vi "VCI_BOARD_INFO_1_CONVERT.vi"(1 "VCI_BOARD_INFO_1":T2) -> (0 "VCI_BOARD_INFO":T1)   [LabVIEW 2018, in "ControlCan.lvlib"]
uses:
  ControlCan.lvlib
  VCI_BOARD_INFO_1.ctl
  VCI_BOARD_INFO.ctl
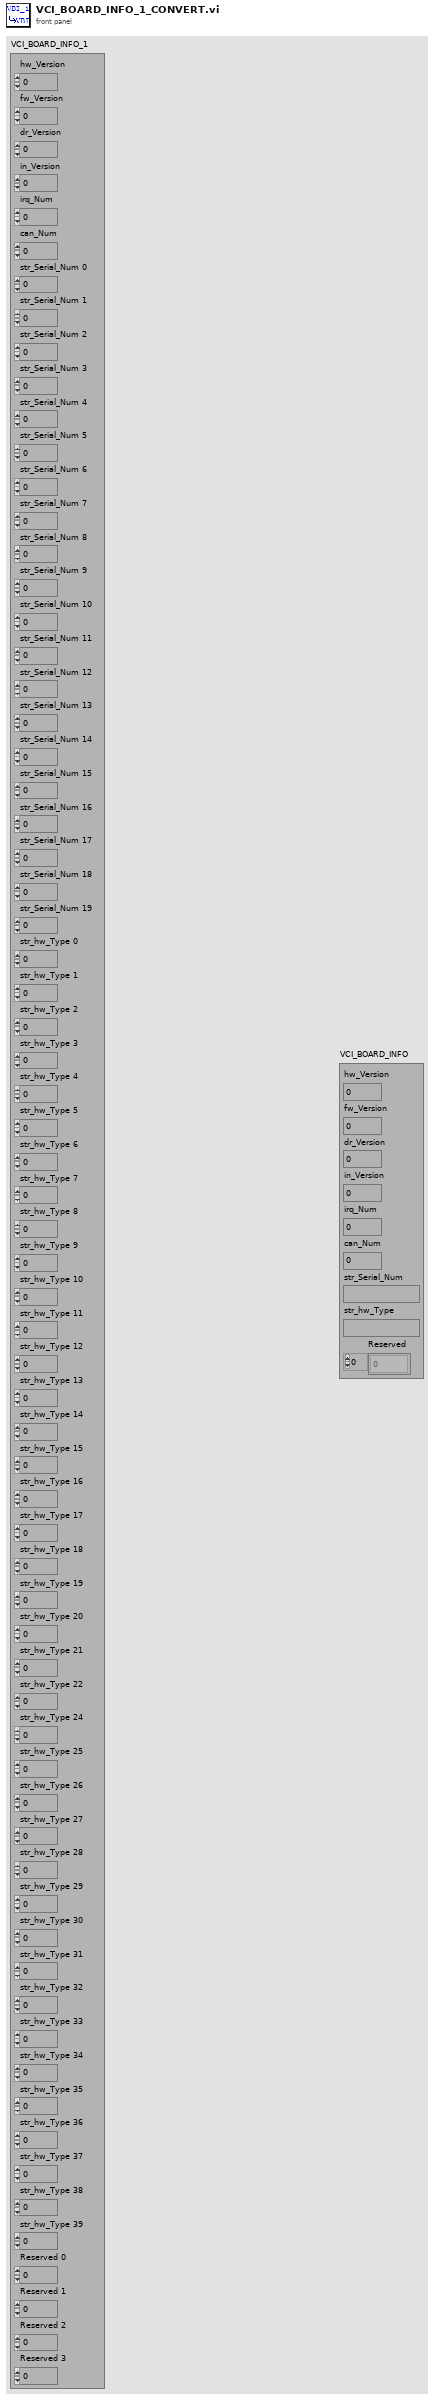
[diagram p1: front panel]
types:
  T1 = typedef "ControlCAN.lvlib/VCI_BOARD_INFO.ctl" = cluster{"hw_Version":u16, "fw_Version":u16, "dr_Version":u16, "in_Version":u16, "irq_Num":u16, "can_Num":u8, "str_Serial_Num":string, "str_hw_Type":string, "Reserved":u8[]}
  T2 = typedef "ControlCAN.lvlib/VCI_BOARD_INFO_1.ctl" = cluster{"hw_Version":u16, "fw_Version":u16, "dr_Version":u16, "in_Version":u16, "irq_Num":u16, "can_Num":u8, "str_Serial_Num 0":u8, "str_Serial_Num 1":u8, "str_Serial_Num 2":u8, "str_Serial_Num 3":u8, "str_Serial_Num 4":u8, "str_Serial_Num 5":u8, "str_Serial_Num 6":u8, "str_Serial_Num 7":u8, "str_Serial_Num 8":u8, "str_Serial_Num 9":u8, "str_Serial_Num 10":u8, "str_Serial_Num 11":u8, "str_Serial_Num 12":u8, "str_Serial_Num 13":u8, "str_Serial_Num 14":u8, "str_Serial_Num 15":u8, "str_Serial_Num 16":u8, "str_Serial_Num 17":u8, "str_Serial_Num 18":u8, "str_Serial_Num 19":u8, "str_hw_Type 0":u8, "str_hw_Type 1":u8, "str_hw_Type 2":u8, "str_hw_Type 3":u8, "str_hw_Type 4":u8, "str_hw_Type 5":u8, "str_hw_Type 6":u8, "str_hw_Type 7":u8, "str_hw_Type 8":u8, "str_hw_Type 9":u8, "str_hw_Type 10":u8, "str_hw_Type 11":u8, "str_hw_Type 12":u8, "str_hw_Type 13":u8, "str_hw_Type 14":u8, "str_hw_Type 15":u8, "str_hw_Type 16":u8, "str_hw_Type 17":u8, "str_hw_Type 18":u8, "str_hw_Type 19":u8, "str_hw_Type 20":u8, "str_hw_Type 21":u8, "str_hw_Type 22":u8, "str_hw_Type 24":u8, "str_hw_Type 25":u8, "str_hw_Type 26":u8, "str_hw_Type 27":u8, "str_hw_Type 28":u8, "str_hw_Type 29":u8, "str_hw_Type 30":u8, "str_hw_Type 31":u8, "str_hw_Type 32":u8, "str_hw_Type 33":u8, "str_hw_Type 34":u8, "str_hw_Type 35":u8, "str_hw_Type 36":u8, "str_hw_Type 37":u8, "str_hw_Type 38":u8, "str_hw_Type 39":u8, "Reserved 0":u8, "Reserved 1":u8, "Reserved 2":u8, "Reserved 3":u8}
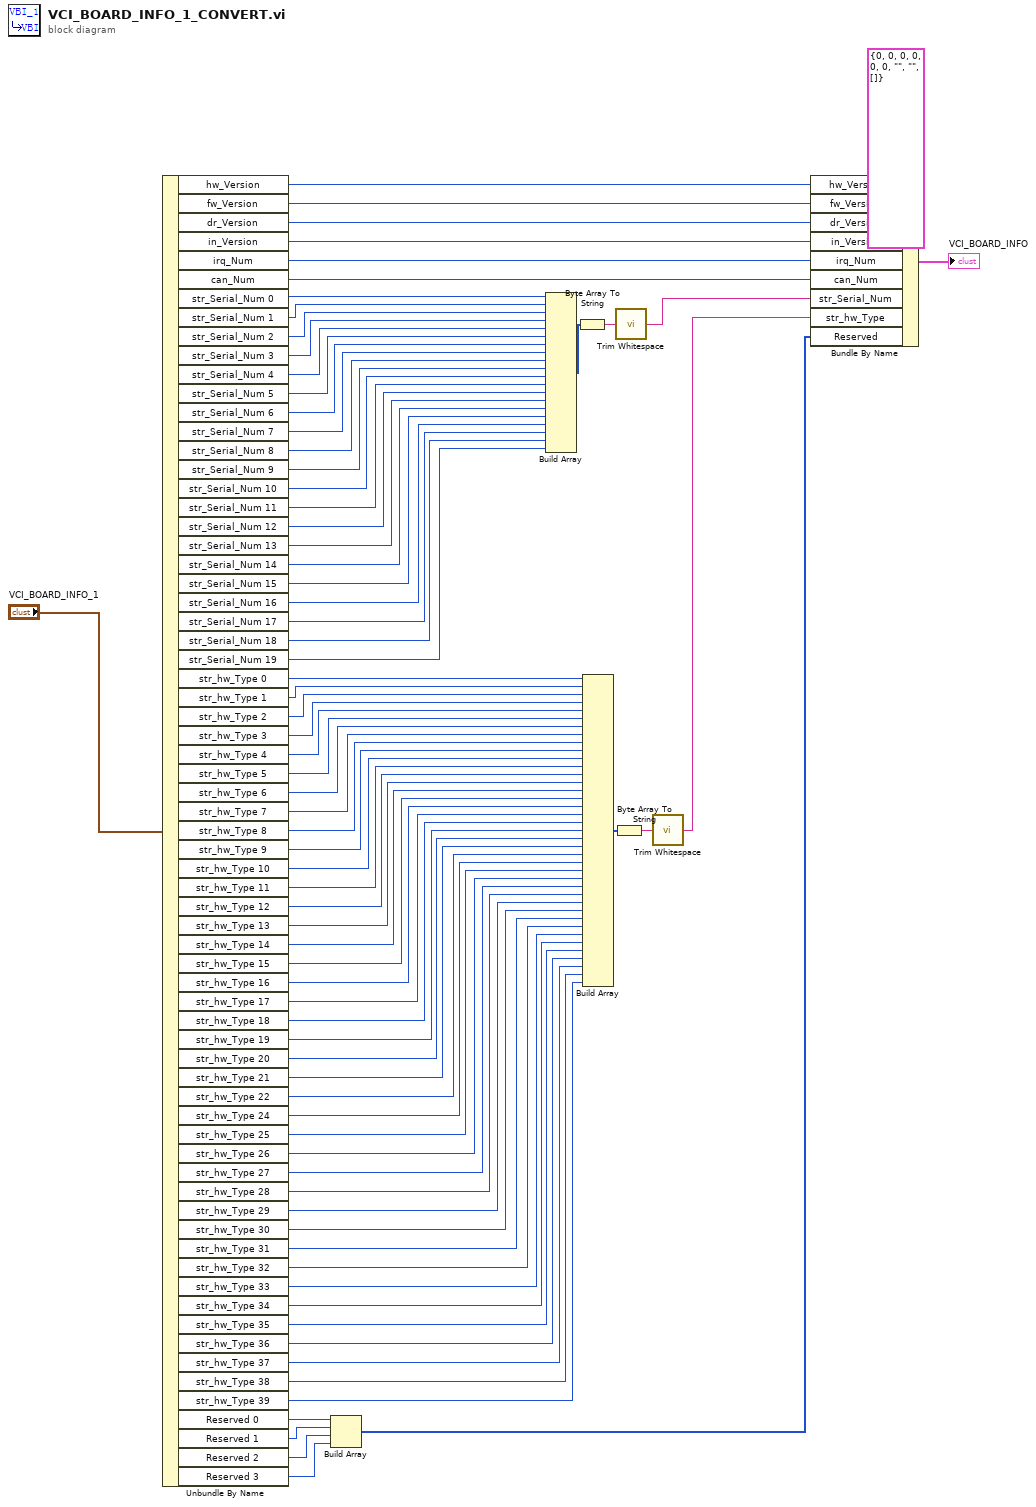
[diagram p0: block diagram]
diagram:
  n1 = Unbundle By Name("VCI_BOARD_INFO_1") -> ("hw_Version"=w77:u16, "fw_Version"=w76:u16, "dr_Version"=w75:u16, "in_Version"=w74:u16, "irq_Num"=w73:u16, "can_Num"=w72:u8, "str_Serial_Num 0"=w71:u8, "str_Serial_Num 1"=w70:u8, "str_Serial_Num 2"=w69:u8, "str_Serial_Num 3"=w68:u8, "str_Serial_Num 4"=w67:u8, "str_Serial_Num 5"=w66:u8, "str_Serial_Num 6"=w65:u8, "str_Serial_Num 7"=w64:u8, "str_Serial_Num 8"=w59:u8, "str_Serial_Num 9"=w58:u8, "str_Serial_Num 10"=w57:u8, "str_Serial_Num 11"=w56:u8, "str_Serial_Num 12"=w55:u8, "str_Serial_Num 13"=w54:u8, "str_Serial_Num 14"=w53:u8, "str_Serial_Num 15"=w52:u8, "str_Serial_Num 16"=w51:u8, "str_Serial_Num 17"=w50:u8, "str_Serial_Num 18"=w49:u8, "str_Serial_Num 19"=w48:u8, "str_hw_Type 0"=w45:u8, "str_hw_Type 1"=w44:u8, "str_hw_Type 2"=w43:u8, "str_hw_Type 3"=w42:u8, "str_hw_Type 4"=w41:u8, "str_hw_Type 5"=w40:u8, "str_hw_Type 6"=w39:u8, "str_hw_Type 7"=w38:u8, "str_hw_Type 8"=w37:u8, "str_hw_Type 9"=w36:u8, "str_hw_Type 10"=w35:u8, "str_hw_Type 11"=w34:u8, "str_hw_Type 12"=w33:u8, "str_hw_Type 13"=w32:u8, "str_hw_Type 14"=w31:u8, "str_hw_Type 15"=w30:u8, "str_hw_Type 16"=w29:u8, "str_hw_Type 17"=w28:u8, "str_hw_Type 18"=w27:u8, "str_hw_Type 19"=w26:u8, "str_hw_Type 20"=w25:u8, "str_hw_Type 21"=w24:u8, "str_hw_Type 22"=w23:u8, "str_hw_Type 24"=w22:u8, "str_hw_Type 25"=w21:u8, "str_hw_Type 26"=w20:u8, "str_hw_Type 27"=w19:u8, "str_hw_Type 28"=w18:u8, "str_hw_Type 29"=w17:u8, "str_hw_Type 30"=w16:u8, "str_hw_Type 31"=w15:u8, "str_hw_Type 32"=w14:u8, "str_hw_Type 33"=w13:u8, "str_hw_Type 34"=w12:u8, "str_hw_Type 35"=w11:u8, "str_hw_Type 36"=w10:u8, "str_hw_Type 37"=w9:u8, "str_hw_Type 38"=w8:u8, "str_hw_Type 39"=w7:u8, "Reserved 0"=w6:u8, "Reserved 1"=w5:u8, "Reserved 2"=w4:u8, "Reserved 3"=w3:u8)
  n2 = Build Array(w6, w5, w4, w3) -> (w1:u8[])
  n3 = Build Array(w71, w70, w69, w68, w67, w66, w65, w64, w59, w58, w57, w56, w55, w54, w53, w52, w51, w50, w49, w48) -> (w63:u8[])
  n4 = Byte Array To String(unsigned byte array=w63) -> (string=w62:string)
  n5 = Build Array(w45, w44, w43, w42, w41, w40, w39, w38, w37, w36, w35, w34, w33, w32, w31, w30, w29, w28, w27, w26, w25, w24, w23, w22, w21, w20, w19, w18, w17, w16, w15, w14, w13, w12, w11, w10, w9, w8, w7) -> (w46:u8[])
  n6 = Byte Array To String(unsigned byte array=w46) -> (string=w47:string)
  n7 = call <vilib>:"Trim Whitespace.vi"("string"=w62) -> ("trimmed string"=w61:string)  [unwired: 1 in]
  n8 = call <vilib>:"Trim Whitespace.vi"("string"=w47) -> ("trimmed string"=w2:string)  [unwired: 1 in]
  n9 = Bundle By Name(cluster=T1 {"hw_Version"=0, "fw_Version"=0, "dr_Version"=0, "in_Version"=0, "irq_Num"=0, "can_Num"=0, "str_Serial_Num"="", "str_hw_Type"="", "Reserved"=[]} ("VCI_BOARD_INFO"), "hw_Version"=w77, "fw_Version"=w76, "dr_Version"=w75, "in_Version"=w74, "irq_Num"=w73, "can_Num"=w72, "str_Serial_Num"=w61, "str_hw_Type"=w2, "Reserved"=w1) -> (→"VCI_BOARD_INFO":T1)
